vi "UpdateFeatureStudio.vi"(6 "did":string, 7 "wid":string, 9 "eid":string, 10 "FeatureScript":string, 11 "Path to creds.json file":path) -> ()   [LabVIEW 2019]
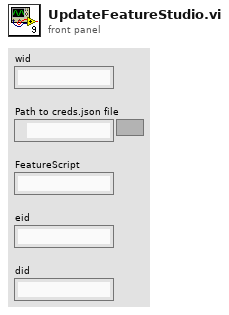
[diagram p1: front panel]
types:
  T1 = cluster{"contents":string, "serializationVersion":string, "sourceMicroversion":string, "rejectMicroversionSkew":bool}
  T2 = cluster{"contents":string, "serializationVersion":string, "sourceMicroversion":string, "rejectMicroversionSkew":bool, "microversionSkew":bool, "libraryVersion":i32}
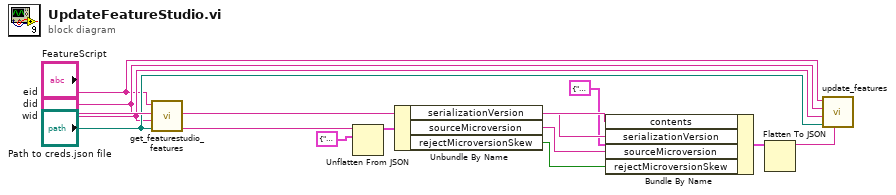
[diagram p0: block diagram]
diagram:
  n1 = call "get_featurestudio_features.vi"("Path to creds.json file"="Path to creds.json file", "wid"="wid", "did"="did", "eid"="eid") -> ("Output Body"=w1:string)  [unwired: 6 in, 1 out]
  n2 = Unflatten From JSON(JSON string=w1, type and defaults=T2 {"contents"="", "serializationVersion"="", "sourceMicroversion"="", "rejectMicroversionSkew"=TRUE, "microversionSkew"=TRUE, "libraryVersion"=0}) -> (value=w10:T2)  [unwired: 5 in, 1 out]
  n3 = Unbundle By Name(w10) -> ("serializationVersion"=w11:string, "sourceMicroversion"=w12:string, "rejectMicroversionSkew"=w13:bool)
  n4 = Bundle By Name(cluster=T1 {"contents"="", "serializationVersion"="", "sourceMicroversion"="", "rejectMicroversionSkew"=TRUE}, "contents"="FeatureScript", "serializationVersion"=w11, "sourceMicroversion"=w12, "rejectMicroversionSkew"=w13) -> (w7:T1)
  n5 = Flatten To JSON(anything=w7) -> (JSON string=w8:string)  [unwired: 2 in, 1 out]
  n6 = call "update_features.vi"("payload"=w8, "Path to creds.json file"="Path to creds.json file", "wid"="wid", "did"="did", "eid"="eid") -> ()  [unwired: 5 in, 2 out]
